vi "Check Admin Identity.vi"(8 "error in (no error)":errorcluster, 10 "UserName(\"\")":string, 11 "Admin_Actor in":refnum<class "Admin_Actor.lvclass">) -> (0 "error out":errorcluster, 2 "CheckIdentity（False）":bool, 3 "Admin_Actor out":refnum<class "Admin_Actor.lvclass">)   [LabVIEW 2015, in "Admin_Actor.lvlib" / "Admin_Actor.lvclass"]
uses:
  Admin_Actor.lvclass
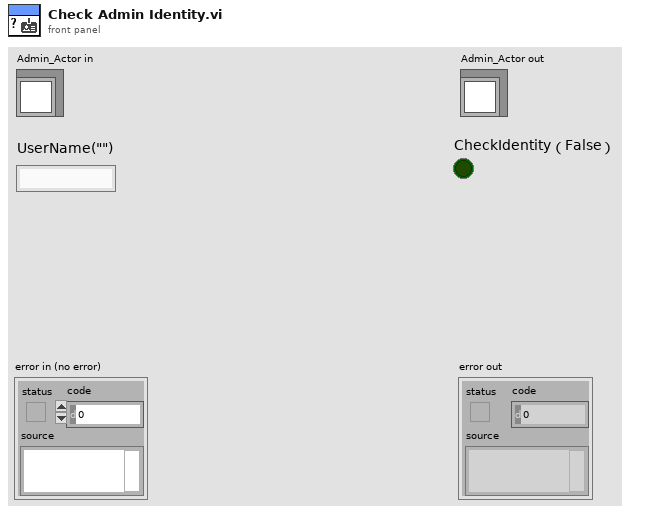
[diagram p1: front panel]
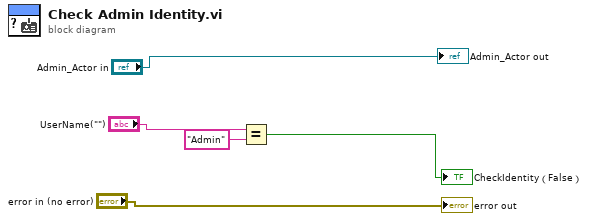
[diagram p0: block diagram]
diagram:
  n1 = Equal?(x="UserName(\"\")", y="Admin") -> (x = y?=→"CheckIdentity（False）":bool)
  "error out" <- "error in (no error)"
  "Admin_Actor out" <- "Admin_Actor in"
